vi "square root.vi"() -> ()   [LabVIEW 2014]
panel:
  out "square root value":dbl
  in  "number":dbl
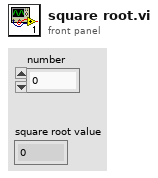
[diagram p1: front panel]
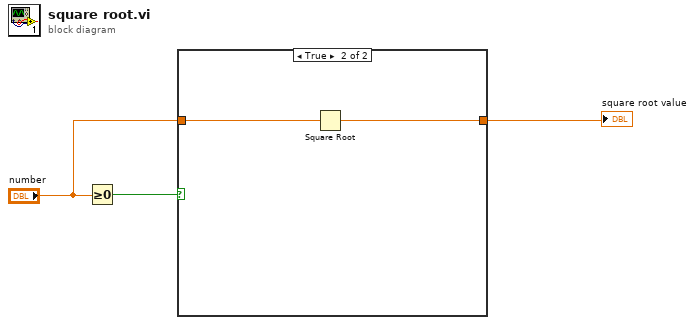
[diagram p0: block diagram]
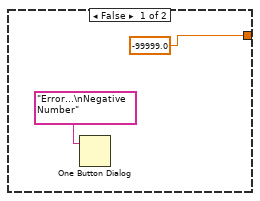
[diagram p2: hidden frame]
diagram:
  n1 = Greater Or Equal To 0?(x="number") -> (x >= 0?=w3:bool)
  n2 = case shown="True" w3 {
    tunnel: "number" -> [_ w7]
    tunnel: [-99999.0 w6] -> w2
    frame False {
      n3 = One Button Dialog(message="Error...\nNegative Number") -> ()  [unwired: 1 in, 1 out]
    }
    frame True {
      n4 = Square Root(x=w7) -> (sqrt(x)=w6:dbl)
    }
  }
  "square root value" <- w2
